vi "Construct Known Types Binder.vi"(5 "Known Types Binder in":refnum<class "Known Types Binder.lvclass">, 8 "error in (no error)":errorcluster, 11 "Known Types":T1[](array[typedef])) -> (0 "error out":errorcluster, 3 "Known Types Binder":refnum<class "Known Types Binder.lvclass">)   [LabVIEW 2017, in "Known Types Binder.lvclass"]
uses:
  Known Types Binder.lvclass
  Known Type.ctl
  Known Types Binder.lvclass/Known Types Binder.ctl
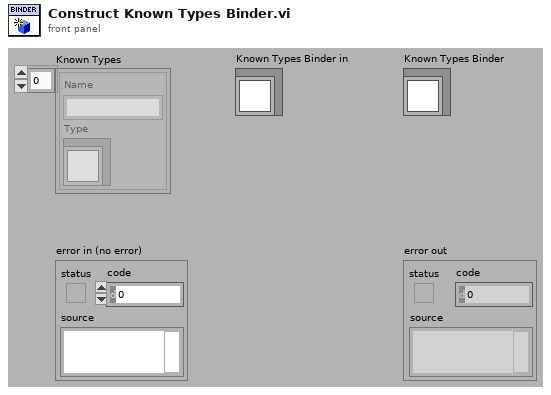
[diagram p1: front panel]
types:
  T1 = typedef "Known Types Binder.lvclass/Known Type.ctl" = cluster{"Name":string, "Type":refnum<class>}
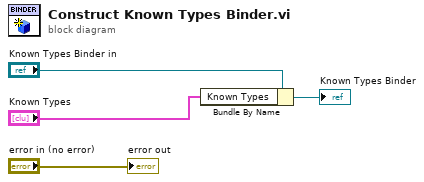
[diagram p0: block diagram]
diagram:
  n1 = Bundle By Name(cluster="Known Types Binder in", "Known Types"="Known Types") -> (→"Known Types Binder":refnum<class "Known Types Binder.lvclass">)
  "error out" <- "error in (no error)"
